vi "check_vlc.vi"(8 "error in (no error)":errorcluster) -> (0 "error out":errorcluster, 1 "Match?":bool, 3 "Open Proceesses":string[](array[string])=["C:\\Program Files\\National Instruments\\LabVIEW 8.2\\LabVIEW.exe"])   [LabVIEW 2018]
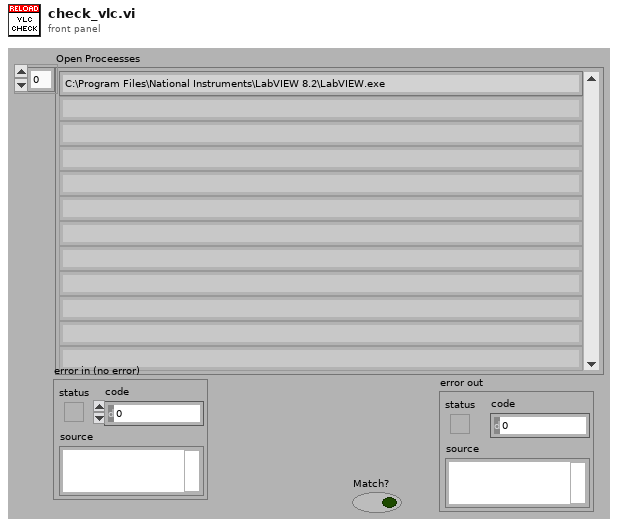
[diagram p1: front panel]
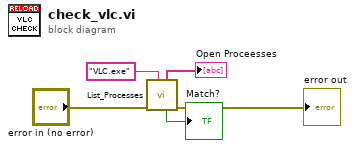
[diagram p0: block diagram]
diagram:
  n1 = call "List_Processes.vi"("Process filter"="VLC.exe", "error in (no error)"="error in (no error)") -> ("error out"=→"error out":errorcluster, "Match?"=→"Match?":bool, "Open Proceesses"=→"Open Proceesses":string[])  [unwired: 7 out]
